vi "Test Set Visible State.vi"(8 "error in (no error)":errorcluster) -> (0 "error out":errorcluster)   [LabVIEW 2020, in "TEST JKI State Machine API.lvlib"]
uses:
  TEST JKI State Machine API.lvlib
  <vilib>/addons/_JKI Toolkits/Caraya/classes/Test/Test.lvclass
  source/JKI SM/JKI SM.lvclass
  <vilib>/addons/_JKI Toolkits/Caraya/classes/Assert/Assert.lvclass
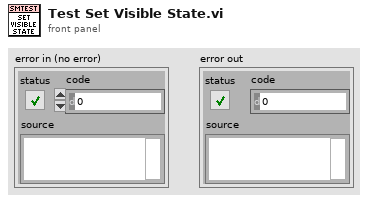
[diagram p1: front panel]
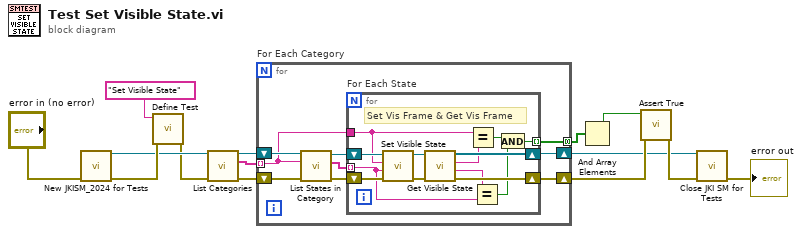
[diagram p0: block diagram]
diagram:
  n1 = call "New JKISM_2024 for Tests.vi"("error in (no error)"="error in (no error)") -> ("error out"=w14:errorcluster, "JKI SM out"=w10:refnum<class "JKI SM.lvclass">)  [unwired: 9 in]
  n2 = call <vilib>:"Define Test.vi"("error in (no error)"=w14, "Label (VI Title)"="Set Visible State") -> ("error out"=w6:errorcluster)  [unwired: 8 in, 1 out]
  n3 = call "List Categories.vi"("error in (no error)"=w6, "JKI SM in"=w10) -> ("error out"=w7:errorcluster, "All State Categories"=w8:string[], "JKI SM out"=w9:refnum<class "JKI SM.lvclass">)  [unwired: 6 in, 1 out]
  n4 = for "For Each Category" {
    tunnel: w8 -> [w16] mode=indexing
    shift-right: [w20] -> w5
    shift-left: w7 -> [w22]
    shift-right: [w18] -> w4
    shift-left: w9 -> [w23]
    tunnel: [w15] -> w3 mode=concatenating
    n5 = call "List States in Category.vi"("error in (no error)"=w22, "Category"=w16, "JKI SM in"=w23) -> ("error out"=w21:errorcluster, "States"=w17:string[], "JKI SM out"=w19:refnum<class "JKI SM.lvclass">)  [unwired: 4 in, 2 out]
    n6 = for "For Each State" {
      shift-right: [w33] -> w20
      shift-left: w21 -> [w36]
      shift-right: [w31] -> w18
      shift-left: w19 -> [w35]
      tunnel: w17 -> [w28] mode=indexing
      tunnel: w16 -> [w29]
      tunnel: [w24] -> w15 mode=indexing
      # "Set Vis Frame & Get Vis Frame"
      n7 = call "Set Visible State.vi"("error in (no error)"=w36, "State Name"=w28, "Category (Optional)"=w29, "JKI SM in"=w35) -> ("error out"=w34:errorcluster, "JKI SM out"=w32:refnum<class "JKI SM.lvclass">)  [unwired: 6 in]
      n8 = call "Get Visible State.vi"("error in (no error)"=w34, "JKI SM in"=w32) -> ("error out"=w33:errorcluster, "State Name"=w27:string, "Category"=w30:string, "JKI SM out"=w31:refnum<class "JKI SM.lvclass">)  [unwired: 4 in, 2 out]
      n9 = Equal?(x=w29, y=w30) -> (x = y?=w26:bool)
      n10 = Equal?(x=w27, y=w28) -> (x = y?=w25:bool)
      n11 = And(x=w26, y=w25) -> (x .and. y?=w24:bool)
    }
  }
  n12 = And Array Elements(Boolean array=w3) -> (logical AND=w2:bool)
  n13 = call <vilib>:"Assert True.vi"("error in (no error)"=w5, "True?"=w2) -> ("error out"=w12:errorcluster)  [unwired: 8 in, 1 out]
  n14 = call "Close JKI SM for Tests.vi"("error in (no error)"=w12, "JKI SM in"=w4) -> ("error out"=→"error out":errorcluster)  [unwired: 9 in]
